vi "algorithm.vi"(10 "String":string) -> (2 "Score":i32)   [LabVIEW 2017]
uses:
  BingoBoard/BingoBoard.lvclass
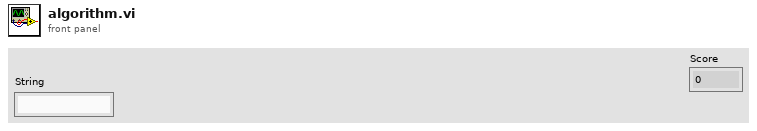
[diagram p1: front panel]
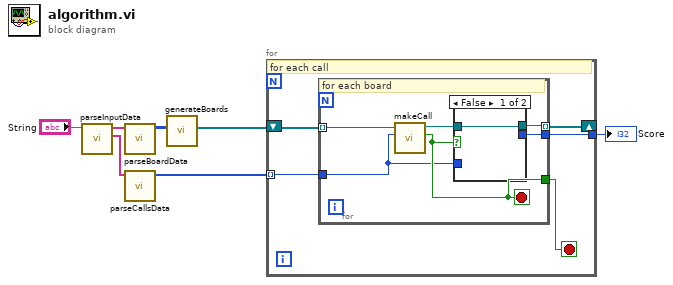
[diagram p0: block diagram]
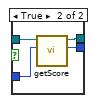
[diagram p2: hidden frame]
diagram:
  n1 = call "parseInputData.vi"("String"="String") -> ("CallsData"=w6:string[], "BoardsData"=w5:string[])  [unwired: 9 in]
  n2 = call "parseBoardData.vi"("Array in"=w5) -> ("Array out"=w4:i32[][][])  [unwired: 10 in]
  n3 = call "parseCallsData.vi"("Array in"=w6) -> ("Array out"=w3:i32[])  [unwired: 10 in]
  n4 = call "generateBoards.vi"("Array"=w4) -> ("BingoBoards"=w2:refnum<class "BingoBoard.lvclass">[])  [unwired: 10 in]
  n5 = for {
    tunnel: w3 -> [w11] mode=indexing
    tunnel: [w9] -> w1
    shift-right: [w8] -> _
    shift-left: w2 -> [w12]
    stop <- w10 stop-if-true
    # "for each call"
    n6 = for {
      tunnel: w12 -> [w18] mode=indexing
      tunnel: w11 -> [w13]
      tunnel: [w17] -> w10
      tunnel: [w15] -> w9
      tunnel: [w14] -> w8 mode=indexing
      stop <- w17 stop-if-true
      # "for each board"
      n7 = call-dynamic "makeCall.vi"("call"=w13, "BingoBoard in"=w18) -> ("won?"=w17:bool, "BingoBoard out"=w16:refnum<class "BingoBoard.lvclass">)  [unwired: 7 in, 1 out]
      n8 = case shown="False" w17 {
        tunnel: w16 -> [w19 w23]
        tunnel: [_ w22] -> w15
        tunnel: [w19 w21] -> w14
        tunnel: w13 -> [_ w20]
        frame False {
        }
        frame True {
          n9 = call-dynamic "getScore.vi"("call"=w20, "BingoBoard in"=w23) -> ("Score"=w22:i32, "BingoBoard out"=w21:refnum<class "BingoBoard.lvclass">)  [unwired: 7 in, 1 out]
        }
      }
    }
  }
  "Score" <- w1
